vi "Exercise 5.vi"() -> ()   [LabVIEW 2017]
panel:
  out "String":string
  in  "Numeric":dbl
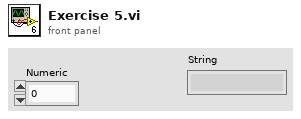
[diagram p1: front panel]
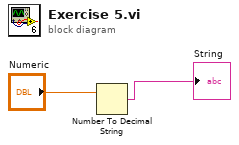
[diagram p0: block diagram]
diagram:
  n1 = Number To Decimal String(number="Numeric") -> (decimal integer string=→"String":string)  [unwired: 1 in]
